vi "LVUSBRH2_VISA_CMD_auto.vi"(8 "error in (no error)":errorcluster caption="error in(no errro)", 9 "auto interval_sec(0)":i32, 11 "VISA rssc":refnum<visa-resource-name>) -> (0 "error out":errorcluster, 3 "VISA rssc out":refnum<visa-resource-name>)   [LabVIEW 2020]
panel:
  out "cmd string":string
  # "0 = off\n10 = 10sec interval"
  # "sec"
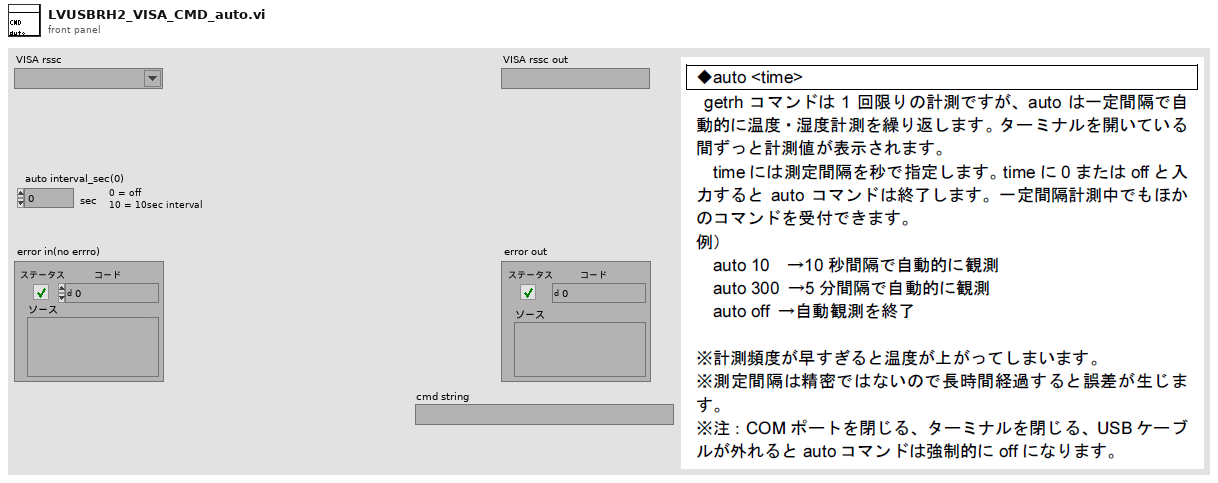
[diagram p1: front panel]
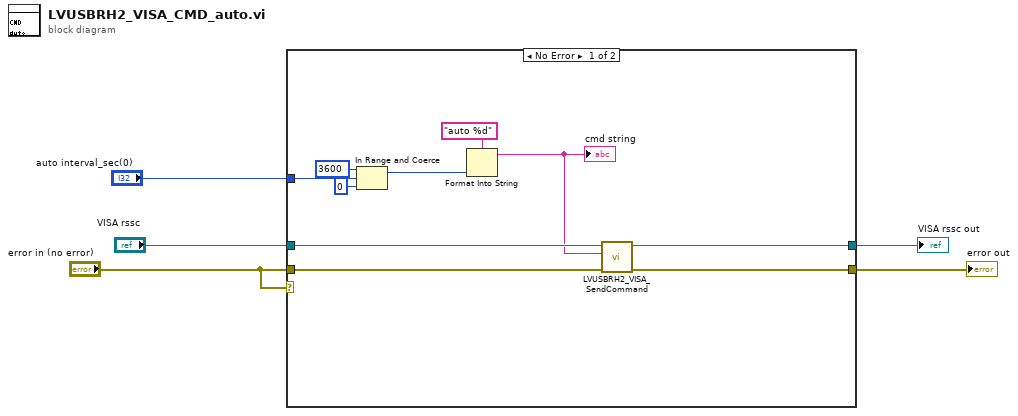
[diagram p0: block diagram]
diagram:
  n1 = case shown="No Error" "error in (no error)" {
    tunnel: "VISA rssc" -> [w15 w17]
    tunnel: [w12 w17] -> w4
    tunnel: "error in (no error)" -> [w13 w16]
    tunnel: [w14 w16] -> w3
    tunnel: "auto interval_sec(0)" -> [w9 _]
    frame No Error {
      n2 = In Range and Coerce(upper limit=3600 ("上限"), x=w9, lower limit=0 ("下限")) -> (coerced(x)=w8:i32)  [unwired: 1 out]
      n3 = Format Into String(format string="auto %d" ("形式文字列"), w8) -> (resulting string=w10:string)  [unwired: 2 in, 1 out]
      "cmd string" <- w10
      n4 = call "LVUSBRH2_VISA_SendCommand.vi"("error in (no error)"=w13, "cmd string"=w10, "VISA rssc"=w15) -> ("error out"=w14:errorcluster, "VISA rssc out"=w12:refnum<visa-resource-name>)  [unwired: 7 in]
    }
    frame Error {
    }
  }
  "VISA rssc out" <- w4
  "error out" <- w3
